vi "get_vector_message_value.vi"(8 "error in (no error)":errorcluster, 11 "message_vectors in":refnum<class "abstract_message_base.lvclass">) -> (0 "error out":errorcluster, 3 "embedding_data":T1[](array[typedef]))   [LabVIEW 2020, in "message_vectors.lvclass"]
uses:
  message_vectors.lvclass
  abstract_message_base/abstract_message_base.lvclass
  embedding.ctl
  message_vectors.lvclass/message_vectors.ctl
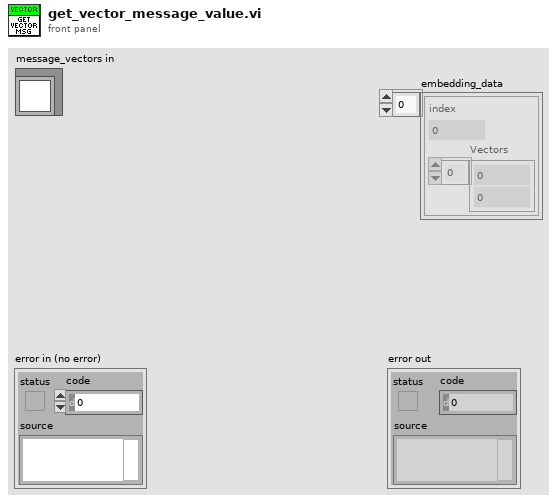
[diagram p1: front panel]
types:
  T1 = typedef "message_vectors.lvclass/embedding.ctl" = cluster{"index":u32, "Vectors":dbl[]}
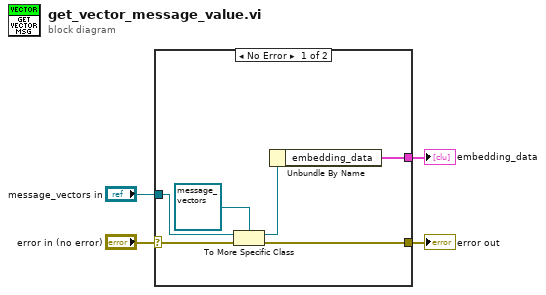
[diagram p0: block diagram]
diagram:
  n1 = case shown="No Error" "error in (no error)" {
    selector: "error in (no error)" -> [w8 w11]
    tunnel: [w7 w11] -> w3
    tunnel: "message_vectors in" -> [w10 _]
    tunnel: [w5 _] -> w1
    frame No Error {
      n2 = To More Specific Class(target class=refnum<class "message_vectors.lvclass"> refnum ("message_vectors.lvclass"), reference=w10, error in=w8) -> (specific class reference=w6:refnum<class "message_vectors.lvclass">, error out=w7:errorcluster)
      n3 = Unbundle By Name(w6) -> ("embedding_data"=w5:T1[])
    }
    frame Error {
    }
  }
  "error out" <- w3
  "embedding_data" <- w1
